vi "Basic 3.vi"() -> ()   [LabVIEW 2014, in "Arduino TFT.lvlib"]
uses:
  <vilib>/Aledyne-TSXperts/Arduino Compatible Compiler for LabVIEW/addons/Arduino TFT/Arduino TFT.lvlib
panel:
  out "Error Out":errorcluster
  in  "Error In":errorcluster
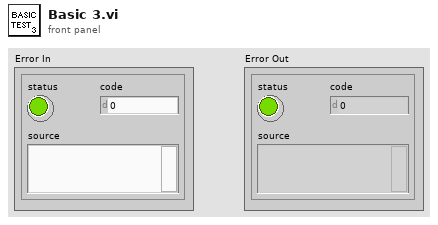
[diagram p1: front panel]
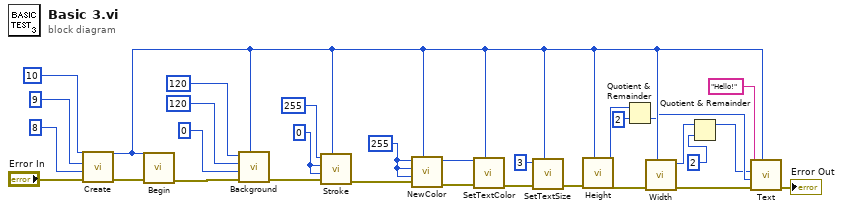
[diagram p0: block diagram]
diagram:
  w18 = u8 255 ("blue")
  w20 = u8 0 ("red")
  n1 = call <vilib>:"Create.vi"("Error In"="Error In", "rst"=u8 8 ("cs"), "rs"=u8 9 ("cs"), "cs"=u8 10) -> ("Error Out"=w26:errorcluster, "Instance"=w7:u32)  [unwired: 4 in]
  n2 = call <vilib>:"Begin.vi"("Error In"=w26, "Instance"=w7) -> ("Error Out"=w25:errorcluster)  [unwired: 8 in]
  n3 = call <vilib>:"Background.vi"("Instance"=w7, "Error In"=w25, "blue"=u8 0 ("red"), "green"=u8 120 ("red"), "red"=u8 120) -> ("Error Out"=w21:errorcluster)  [unwired: 6 in]
  n4 = call <vilib>:"Stroke.vi"("Instance"=w7, "Error In"=w21, "blue"=w20, "green"=w20, "red"=u8 255) -> ("Error Out"=w11:errorcluster)  [unwired: 6 in]
  n5 = call <vilib>:"NewColor.vi"("Instance"=w7, "Error In"=w11, "blue"=w18, "green"=w18, "red"=w18) -> ("Error Out"=w17:errorcluster, "color"=w16:u16)  [unwired: 5 in]
  n6 = call <vilib>:"SetTextColor.vi"("Instance"=w7, "Error In"=w17, "color"=w16) -> ("Error Out"=w13:errorcluster)  [unwired: 8 in]
  n7 = call <vilib>:"SetTextSize.vi"("Instance"=w7, "Error In"=w13, "size"=u8 3) -> ("Error Out"=w8:errorcluster)  [unwired: 8 in]
  n8 = call <vilib>:"Height.vi"("Instance"=w7, "Error In"=w8) -> ("Error Out"=w9:errorcluster, "height"=w6:i16)  [unwired: 8 in]
  n9 = Quotient & Remainder(x=w6, y=i16 2) -> (floor(x/y)=w2:i16)  [unwired: 1 out]
  n10 = call <vilib>:"Width.vi"("Instance"=w7, "Error In"=w9) -> ("Error Out"=w10:errorcluster, "height"=w4:i16)  [unwired: 8 in]
  n11 = Quotient & Remainder(x=w4, y=i16 2) -> (x-y*floor(x/y)=w1:i16)  [unwired: 1 out]
  n12 = call <vilib>:"Text.vi"("Instance"=w7, "Error In"=w10, "y"=w2, "x"=w1, "text"="Hello!") -> ("Error Out"=→"Error Out":errorcluster)  [unwired: 6 in]
